vi "Tokenize String.vi"(4 "delimiter ([\\s\\t\\n\\r]+)":string="[ \t\n\r]+", 5 "input string":string) -> (0 "token array":string[](array[string]), 2 "number of tokens":i32)   [LabVIEW 2012, in "TLB` Template.lvlib" / "Tools_String.lvlib"]
doc: "Separates input string into an array of substrings. Delimiter specifies what separates the substrings.\n\nCharacters that are preceded by a '\\' are not matched with delimiter.\n\nExample:\ndelimiter=\"[ ]+\" (i.e. one or more spaces)\ninput string= \"hello world foo\\ bar\"\n\ntoken array=[\"hello\",\"world\",\"foo bar\"]"
uses:
  Tools_String.lvlib
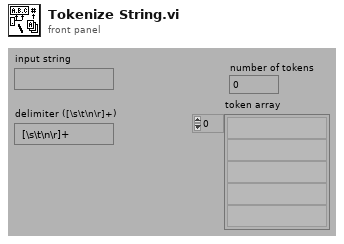
[diagram p1: front panel]
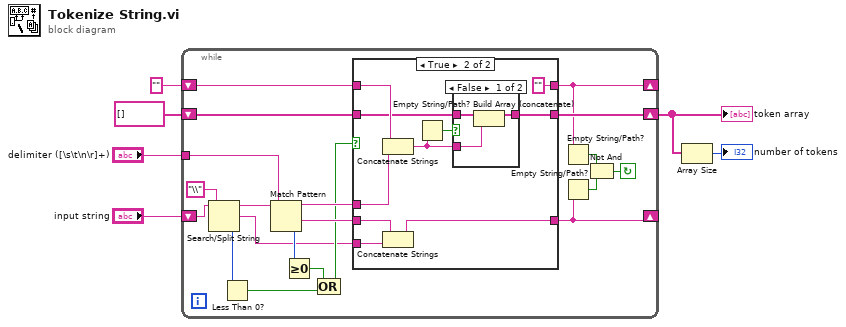
[diagram p0: block diagram]
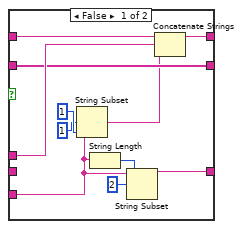
[diagram p2: hidden frame]
diagram:
  n1 = while {
    shift-left: "" ("before substring") -> [w22]
    shift-right: [w16] -> _
    shift-left: string[] [] -> [w25]
    shift-right: [w24] -> w3
    shift-left: "input string" -> [w11]
    shift-right: [w19] -> _
    tunnel: "delimiter ([\\s\\t\\n\\r]+)" -> [w26]
    stop <- w13 continue-if-true
    n2 = Search/Split String(string=w11, search string/char (-)="\\" ("search char (-)")) -> (substring before match=w9:string, match + rest of string=w8:string, offset of match=w10:i32)  [unwired: 1 out]
    n3 = Less Than 0?(x=w10) -> (x < 0?=w12:bool)
    n4 = Match Pattern(string=w9, regular expression=w26) -> (before substring=w23:string, after substring=w21:string, offset past match=w20:i32)  [unwired: 2 out]
    n5 = Greater Or Equal To 0?(x=w20) -> (x >= 0?=w18:bool)
    n6 = Compound Arithmetic op=OR(w18, w12) -> (w17:bool)
    n7 = case shown="True" w17 {
      tunnel: w23 -> [w36 w42]
      tunnel: [w34 w45] -> w24
      tunnel: w25 -> [w34 w44]
      tunnel: w22 -> [w37 w46]
      tunnel: w21 -> [_ w40]
      tunnel: [w30 w39] -> w19
      tunnel: [w35 ""] -> w16
      tunnel: w8 -> [w27 w38]
      frame False {
        n8 = String Subset(string=w27, offset (0)=1 ("length"), length (rest)=1 ("length")) -> (substring=w29:string)
        n9 = String Length(string=w27) -> (length=w31:i32)
        n10 = String Subset(string=w27, offset (0)=2, length (rest)=w31) -> (substring=w30:string)
        n11 = Concatenate Strings(w37, w36, w29) -> (w35:string)
      }
      frame True {
        n12 = Concatenate Strings(w46, w42) -> (w47:string)
        n13 = Concatenate Strings(w40, w38) -> (w39:string)
        n14 = Empty String/Path?(string/path=w47) -> (empty?=w43:bool)
        n15 = case shown="False" w43 {
          tunnel: w44 -> [w50 w51]
          tunnel: [w49 w51] -> w45
          tunnel: w47 -> [w48 _]
          frame False {
            n16 = Build Array (concatenate)(w50, w48) -> (w49:string[])
          }
          frame True {
          }
        }
      }
    }
    n17 = Empty String/Path?(string/path=w16) -> (empty?=w15:bool)
    n18 = Empty String/Path?(string/path=w19) -> (empty?=w14:bool)
    n19 = Not And(1:w14, 2:w15) -> (0:w13:bool)
  }
  "token array" <- w3
  n20 = Array Size(array=w3) -> (size(s)=→"number of tokens":i32)
